vi "Test Draw ARGB With Mask.vi"(8 "error in (no error)":errorcluster, 11 "Test Case In":refnum<class "Image.lvclass">) -> (0 "error out":errorcluster, 3 "Test Case Out":refnum<class "Image.lvclass">)   [LabVIEW 2020, in "test.lvlib" / "Image.lvclass"]
uses:
  Image.lvclass
  C:/Program Files (x86)/National Instruments/LabVIEW 2020/vi.lib/Astemes/LUnit/Test Case.lvclass
  common/Image Size (Integer).ctl
  <vilib>/Astemes/LUnit/Test Case.lvclass/Test Case.ctl
  image/New Image (ARGB).vi
  image/New Image (Greyscale).vi
  image/Copy Pixmap to Image (ARGB with Mask Output).vi
  image/Draw Image to Picture (ARGB with Mask).vi
  4993e8ee-a06a-463a-9684-69129f64d5ce.vi
  image/Copy Array to Image.vi
  image/Copy Array to Image (ARGB).vi
  image/New Image (ARGB).vi/3321fa97-f432-4e1e-8db9-a0df79aed21b.vi
  image/ARGB Colour to U32 Pixel Value.vi
  image/New Image (Greyscale).vi/6598b9e0-8a08-46f5-91fd-ca1b87217137.vi
  image/Copy Pixmap to Image (ARGB with Mask Output).vi/a116197e-b340-4968-94fb-08de404a21d3.vi
  image/Draw Image to Picture (ARGB with Mask).vi/8cd07b1b-062e-4fe4-9e87-2eb3dc89fe0e.vi
  <vilib>/Astemes/LUnit/Append Pass Result.vi
  <vilib>/Astemes/LUnit/Append Fail Result.vi
  <vilib>/Astemes/LUnit/Describe Comparison.vi
  4993e8ee-a06a-463a-9684-69129f64d5ce.vi/9c5d11cd-9439-4240-a1ee-d9baace9c924.vi
  image/FixPixmap.vi
  <vilib>/Astemes/LUnit/Run In UI.vi
  image/Default8bitColourMap.vi
  <vilib>/Utility/error.llb/Clear Errors.vi
  common/Module Path.vi
  <vilib>/Utility/error.llb/Error Cluster From Error Code.vi
  <vilib>/picture/pixmap.llb/Flatten Pixmap.vi
  <vilib>/Astemes/LUnit/Describe Variant.vi
  image/image.lvlib
  common/common.lvlib
panel:
  out "Actual":picture
  out "Expected":picture
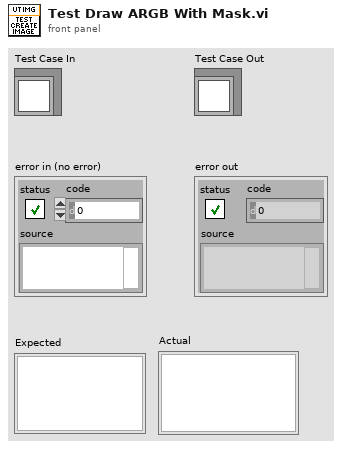
[diagram p1: front panel]
types:
  T1 = typedef "common.lvlib/Image Size (Integer).ctl" = cluster{"Width":u16, "Height":u16}
  T2 = typedef "imagedata.ctl" = cluster{"image type":i32, "image depth":i32, "image":u8[], "mask":u8[], "colors":u32[], "Rectangle":cluster{"left":i16, "top":i16, "right":i16, "bottom":i16}}
  T3 = typedef "image.lvlib/ARGB Image.ctl" = refnum<data-value>
  T4 = typedef "image.lvlib/Greyscale Image.ctl" = refnum<data-value>
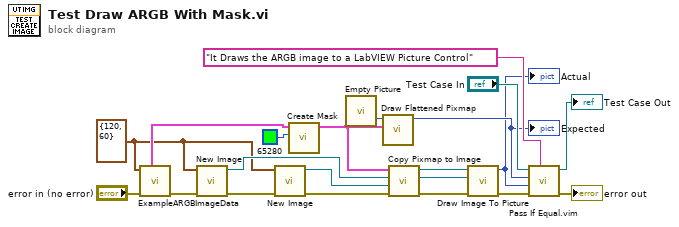
[diagram p0: block diagram]
diagram:
  w8 = T1 {"Width"=120, "Height"=60} ("Preallocated Image Size (Default - 0,0)")
  n1 = call "ExampleARGBImageData.vi"("error in (no error)"="error in (no error)", "Image Size"=w8) -> ("error out"=w4:errorcluster, "ARGB Pixmap Data"=w14:T2)  [unwired: 6 in, 2 out]
  n2 = call-poly "New Image.vi"("error in (no error)"=w4, "Preallocated Image Size (Default: 0,0)"=w8) -> ("error out"=w2:errorcluster, "New ARGB Image"=w12:T3)  [unwired: 8 in]
  n3 = call-poly "New Image.vi"("error in (no error)"=w2, "Preallocated Image Size (Default 0,0)"=w8) -> ("error out"=w1:errorcluster, "New Greyscale Image"=w11:T4)  [unwired: 8 in]
  n4 = call <vilib>:"Create Mask.vi"("Mask Color (Black)"=u32 65280, "image data"=w14) -> ("image data"=w9:T2)  [unwired: 9 in]
  n5 = call "Empty Picture"() -> ("empty picture"=w17:picture)
  n6 = call <vilib>:"Draw Flattened Pixmap.vi"("image data"=w9, "picture"=w17) -> ("new picture"=w16:picture)  [unwired: 7 in]
  "Expected" <- w16
  n7 = call-poly "Copy Pixmap to Image.vi"("error in (no error)"=w1, "Greyscale Image Mask"=w11, "ARGB Image Destination"=w12, "Pixmap Image Data"=w9) -> ("error out"=w10:errorcluster, "Greyscale Image Mask (duplicate)"=w6:T4, "ARGB Image Destination (duplicate)"=w7:T3)  [unwired: 5 in]
  n8 = call-poly "Draw Image To Picture.vi"("error in (no error)"=w10, "Greyscale Mask"=w6, "ARGB Image Source"=w7) -> ("error out"=w5:errorcluster, "Picture"=w15:picture)  [unwired: 7 in]
  "Actual" <- w15
  n9 = call "Pass If Equal.vim"("Description"="It Draws the ARGB image to a LabVIEW Picture Control", "error in (no error)"=w5, "Actual"=w15, "Expected"=w16, "LUnit Test Case In"="Test Case In") -> ("error out"=→"error out":errorcluster, "LUnit Test Case Out"=→"Test Case Out":refnum<class "Image.lvclass">)  [unwired: 5 in]
